vi "Ramping.vi"(5 "SecondaryRamping":dbl, 7 "PrimaryRamping":dbl, 9 "Right Power":dbl, 10 "Left Power":dbl) -> (0 "Right Secondary":dbl, 1 "Right Primary":dbl, 2 "Left Secondary":dbl, 3 "Left Primary":dbl)   [LabVIEW 2014]
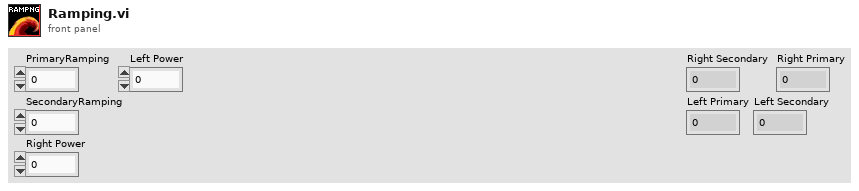
[diagram p1: front panel]
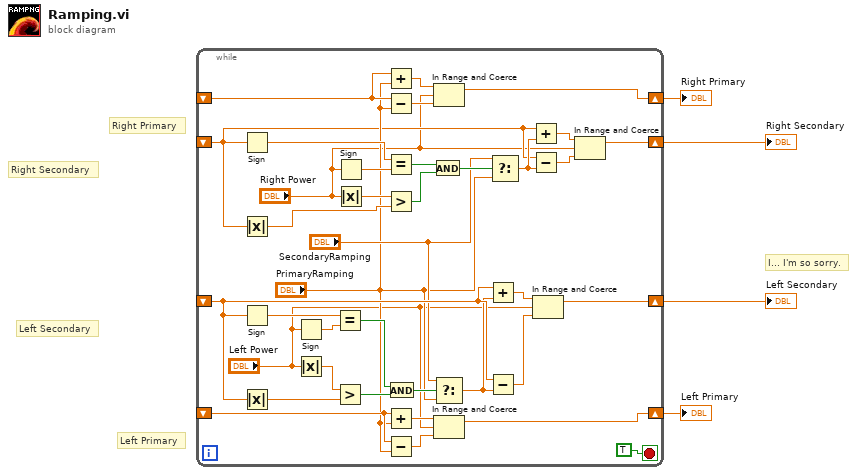
[diagram p0: block diagram]
diagram:
  # "I... I'm so sorry."
  # "Right Secondary"
  # "Right Primary"
  # "Left Secondary"
  # "Left Primary"
  n1 = while {
    shift-right: [w33] -> w3
    shift-left: _ -> [w21]
    shift-right: [w32] -> w2
    shift-left: _ -> [w20]
    shift-right: [w31] -> w1
    shift-left: _ -> [w29]
    shift-right: [w30] -> w4
    shift-left: _ -> [w8]
    stop <- TRUE stop-if-true
    n2 = Sign(1:w8) -> (0:w18:dbl)
    n3 = Absolute Value(x=w8) -> (abs(x)=w15:dbl)
    n4 = Sign(1:w20) -> (0:w22:dbl)
    n5 = Absolute Value(x=w20) -> (abs(x)=w27:dbl)
    n6 = Sign(1:"Left Power") -> (0:w24:dbl)
    n7 = Absolute Value(x="Left Power") -> (abs(x)=w25:dbl)
    n8 = Equal?(x=w22, y=w24) -> (x = y?=w23:bool)
    n9 = Greater?(x=w25, y=w27) -> (0:w26:bool)
    n10 = Sign(1:"Right Power") -> (0:w17:dbl)
    n11 = Absolute Value(x="Right Power") -> (abs(x)=w16:dbl)
    n12 = Add(x=w29, y="PrimaryRamping") -> (x+y=w37:dbl)
    n13 = Subtract(x=w29, y="PrimaryRamping") -> (x-y=w36:dbl)
    n14 = Equal?(x=w18, y=w17) -> (x = y?=w14:bool)
    n15 = Greater?(x=w16, y=w15) -> (0:w13:bool)
    n16 = Add(x=w21, y="PrimaryRamping") -> (x+y=w41:dbl)
    n17 = Subtract(x=w21, y="PrimaryRamping") -> (x-y=w40:dbl)
    n18 = And(x=w23, y=w26) -> (x .and. y?=w28:bool)
    n19 = And(x=w14, y=w13) -> (x .and. y?=w12:bool)
    n20 = In Range and Coerce(upper limit=w37, x="Right Power", lower limit=w36) -> (coerced(x)=w31:dbl)  [unwired: 1 out]
    n21 = Select(t="SecondaryRamping", s=w28, f="PrimaryRamping") -> (s? t:f=w19:dbl)
    n22 = In Range and Coerce(upper limit=w41, x="Left Power", lower limit=w40) -> (coerced(x)=w33:dbl)  [unwired: 1 out]
    n23 = Add(x=w20, y=w19) -> (x+y=w38:dbl)
    n24 = Subtract(x=w20, y=w19) -> (x-y=w39:dbl)
    n25 = Select(t="SecondaryRamping", s=w12, f="PrimaryRamping") -> (s? t:f=w9:dbl)
    n26 = Add(x=w8, y=w9) -> (x+y=w34:dbl)
    n27 = Subtract(x=w8, y=w9) -> (x-y=w35:dbl)
    n28 = In Range and Coerce(upper limit=w38, x="Left Power", lower limit=w39) -> (coerced(x)=w32:dbl)  [unwired: 1 out]
    n29 = In Range and Coerce(upper limit=w34, x="Right Power", lower limit=w35) -> (coerced(x)=w30:dbl)  [unwired: 1 out]
  }
  "Right Secondary" <- w4
  "Left Primary" <- w3
  "Left Secondary" <- w2
  "Right Primary" <- w1
